vi "CUIT553_command_string_driver.vi"(5 "command":T1, 6 "00/01":string, 7 "adress":i32, 8 "Error In":errorcluster) -> (0 "Error Out":errorcluster, 2 "Command":string, 4 "comand out":string)   [LabVIEW 2018]
uses:
  CUIT553_COMMANDs_driver.ctl
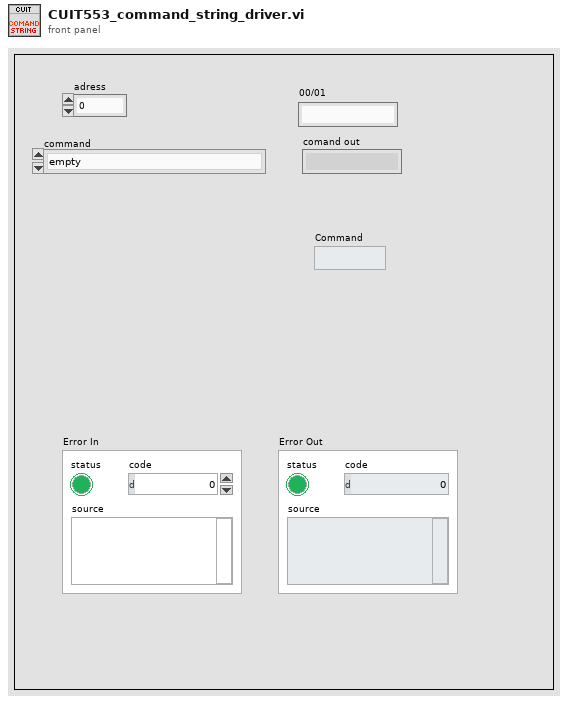
[diagram p1: front panel]
types:
  T1 = typedef "CUIT553_COMMANDs_driver.ctl" = enum16{"empty", "INIT", "T1T2", "T2T3", "T3T4", "T4T5", "T5P1", "P1P2", "P2P3", "P3", "ROUNDS", "RPM", "RESET", "DRAIN READ", "DRAIN CONTROL"}
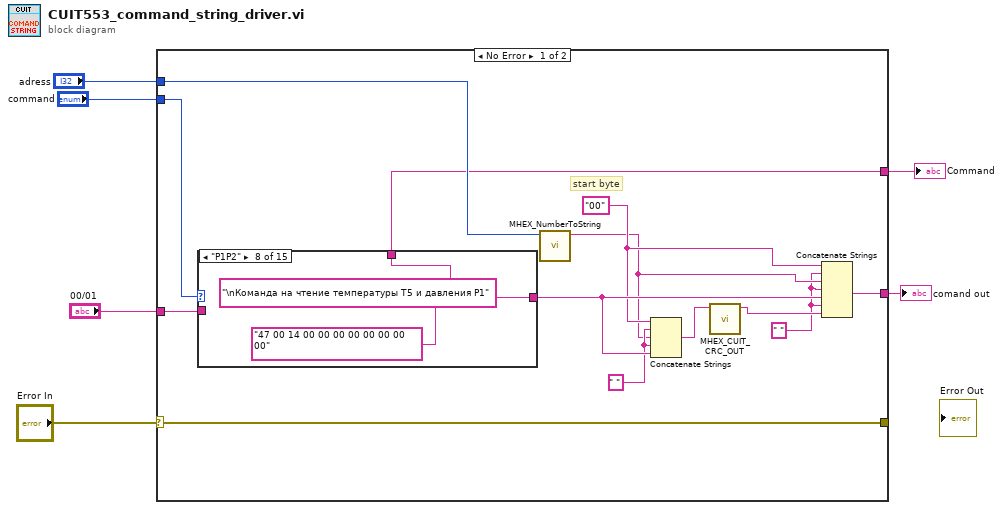
[diagram p0: block diagram]
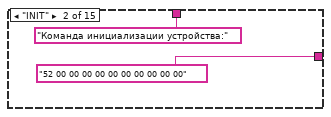
[diagram p3: hidden frame]
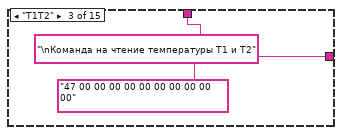
[diagram p4: hidden frame]
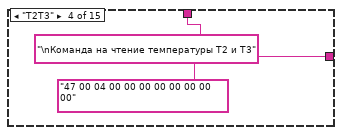
[diagram p5: hidden frame]
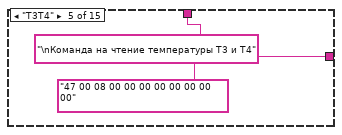
[diagram p6: hidden frame]
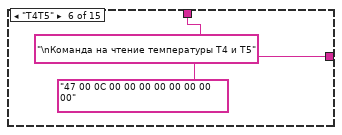
[diagram p7: hidden frame]
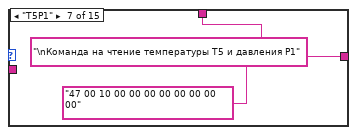
[diagram p8: hidden frame]
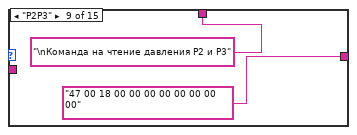
[diagram p9: hidden frame]
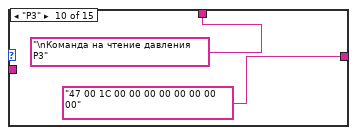
[diagram p10: hidden frame]
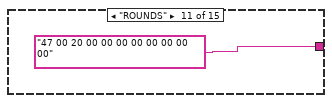
[diagram p11: hidden frame]
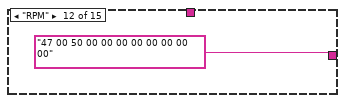
[diagram p12: hidden frame]
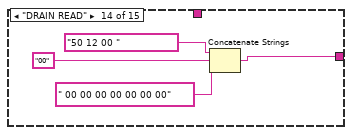
[diagram p14: hidden frame]
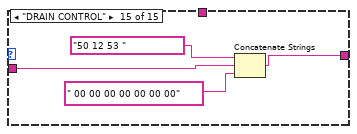
[diagram p15: hidden frame]
diagram:
  n1 = case shown="No Error" "Error In" {
    selector: "Error In" -> [w16 w48]
    tunnel: "adress" -> [w19 _]
    tunnel: [w17 _] -> w5
    tunnel: [w16 w48] -> _
    tunnel: "command" -> [w15 _]
    tunnel: "00/01" -> [w14 _]
    tunnel: [w7 _] -> w2
    frame No Error {
      w11 = " "
      w8 = " " ("string")
      w10 = "00"
      # "start byte"
      n2 = case shown="\"P1P2\"" w15 {
        tunnel: [_ "52 00 00 00 00 00 00 00 00 00 00" ("STRING HEX") "47 00 00 00 00 00 00 00 00 00 00" ("STRING HEX") "47 00 04 00 00 00 00 00 00 00 00" ("STRING HEX") "47 00 08 00 00 00 00 00 00 00 00" ("STRING HEX") "47 00 0C 00 00 00 00 00 00 00 00" ("STRING HEX") "47 00 10 00 00 00 00 00 00 00 00" ("STRING HEX") "47 00 14 00 00 00 00 00 00 00 00" ("STRING HEX") "47 00 18 00 00 00 00 00 00 00 00" ("STRING HEX") "47 00 1C 00 00 00 00 00 00 00 00" ("STRING HEX") "47 00 20 00 00 00 00 00 00 00 00" ("STRING HEX") "47 00 50 00 00 00 00 00 00 00 00" ("STRING HEX") _ w41 w45] -> w12
        tunnel: w14 -> [_ _ _ _ _ _ _ _ _ _ _ _ _ _ w44]
        tunnel: [_ "Команда инициализации устройства:" "\nКоманда на чтение температуры T1 и T2" "\nКоманда на чтение температуры T2 и T3" "\nКоманда на чтение температуры T3 и T4" "\nКоманда на чтение температуры T4 и T5" "\nКоманда на чтение температуры T5 и давления P1" "\nКоманда на чтение температуры T5 и давления P1" "\nКоманда на чтение давления P2 и P3" "\nКоманда на чтение давления P3" _ _ _ _ _] -> w7
        frame "empty", Default {
        }
        frame "INIT" {
        }
        frame "T1T2" {
        }
        frame "T2T3" {
        }
        frame "T3T4" {
        }
        frame "T4T5" {
        }
        frame "T5P1" {
        }
        frame "P1P2" {
        }
        frame "P2P3" {
        }
        frame "P3" {
        }
        frame "ROUNDS" {
        }
        frame "RPM" {
        }
        frame "RESET" {
        }
        frame "DRAIN READ" {
          n3 = Concatenate Strings("50 12 00 " ("STRING HEX"), "00" ("string"), " 00 00 00 00 00 00 00" ("STRING HEX")) -> (w41:string)
        }
        frame "DRAIN CONTROL" {
          n4 = Concatenate Strings("50 12 53 " ("STRING HEX"), w44, " 00 00 00 00 00 00 00" ("STRING HEX")) -> (w45:string)
        }
      }
      n5 = call "MHEX_NumberToString.vi"("Number"=w19) -> ("Result string"=w9:string)  [unwired: 10 in]
      n6 = Concatenate Strings(w10, w11, w9, w11, w12) -> (w18:string)
      n7 = call "MHEX_CUIT_CRC_OUT.vi"("String"=w18) -> ("hex integer string"=w13:string)  [unwired: 9 in, 1 out]
      n8 = Concatenate Strings(w10, w8, w9, w8, w12, w8, w13) -> (w17:string)
    }
    frame Error {
    }
  }
  "comand out" <- w5
  "Command" <- w2
